vi "demo - math to file.vi"() -> ()   [LabVIEW 2024]
doc: "#vi_description \nPlots a polynomial equation to an XY graph and stores the values into a text file.\nThetic Engineering Ltd."
uses:
  <vilib>/Utility/sysdir.llb/System Directory Type.ctl
panel:
  in  "All data":dbl[][](array[numeric])=[[-10.0, -204.0, 492.55], [-9.0, -132.17359, 359.580355], [-8.0, -87.56192, 252.88208], [-7.0, -58.99533, 169.671655], [-6.0, -39.66976, 107.11768], [-5.0, -25.71875, 62.346875], [-4.0, -15.13824, 32.45008], [-3.0, -7.01377, 14.488255], [-2.0, -0.99968, 5.49848], [-1.0, 3.00009, 2.499955], [0.0, 5.0, 2.5], [1.0, 5.00011, 2.500055], [2.0, 3.00288, -0.49832], [3.0, -0.97003, -9.487445], [4.0, -6.81056, -27.44752], [5.0, -14.15625, -57.340625], [6.0, -22.07104, -102.10472], [7.0, -28.52447, -164.647645], [8.0, -29.61888, -247.84112], [9.0, -18.51421, -354.514745]]
  out "XY Graph":cluster{"x axis":dbl[], "plot 1":dbl[]}[](graph)
  out "Data written to":path
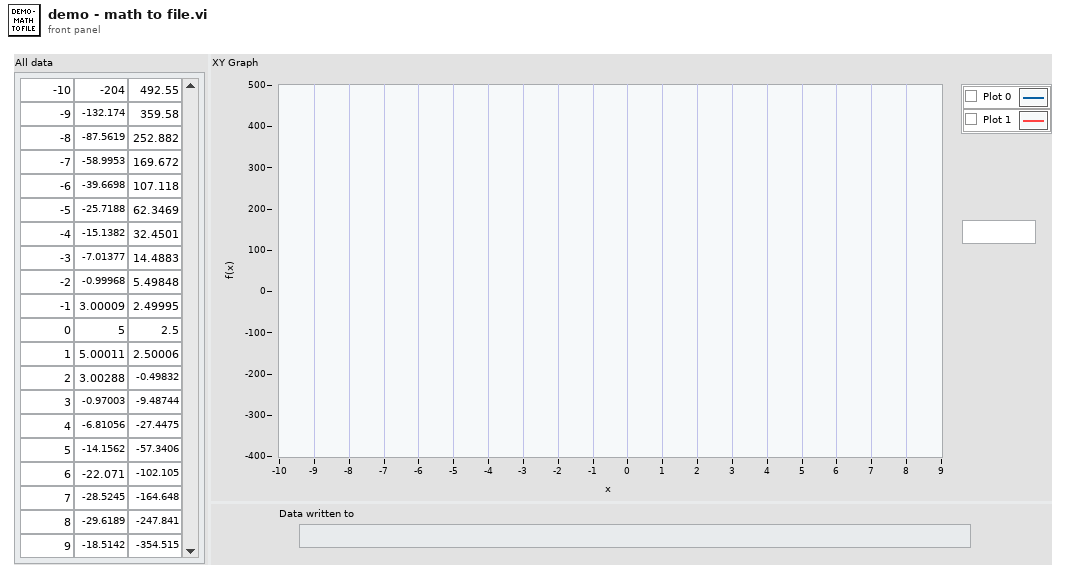
[diagram p1: front panel]
types:
  T1 = enum16{"open", "replace", "create", "open or create", "replace or create", "replace or create with confirmation"}
  T2 = typedef "System Directory Type.ctl" = i32
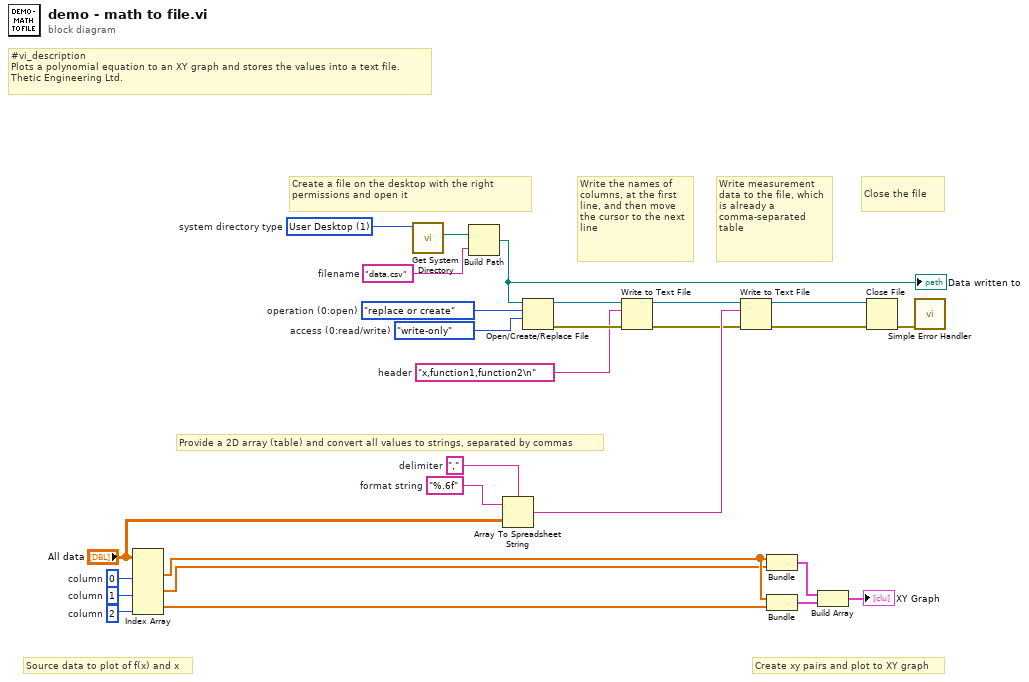
[diagram p0: block diagram]
diagram:
  w5 = 2  # column
  w6 = 1  # column
  w7 = 0  # column
  w9 = "x,function1,function2\n"  # header
  w11 = "data.csv"  # filename
  w12 = enum16{"read/write", "read-only", "write-only"}."write-only"  # access (0:read/write)
  w13 = T1."replace or create"  # operation (0:open)
  w15 = T2 1 items=["User Home"=0, "User Desktop"=1, "User Documents"=2, "User Application Data"=3, "User Preferences"=4, "User Temporary"=5, "Public Documents"=6, "Public Application Data"=7, "Public Preferences"=8, "Public Cache"=13, "System Core Libraries"=9, "System Installed Libraries"=10, "Application Files"=11, "Boot Volume Root"=12]  # system directory type
  w23 = ","  # delimiter
  w24 = "%.6f"  # format string
  # "Close the file"
  # "Write measurement data to the file, which is already a comma-separated table"
  # "Write the names of columns, at the first line, and then move the cursor to the next line"
  # "Create a file on the desktop with the right permissions and open it"
  # "Provide a 2D array (table) and convert all values to strings, separated by commas"
  # "Source data to plot of f(x) and x"
  # "#vi_description \nPlots a polynomial equation to an XY graph and stores the values into a text file.\nThetic Engineering Ltd."
  # "Create xy pairs and plot to XY graph"
  n1 = Index Array(array="All data", index (col) #1=w7, index (col) #2=w6, index (col) #3=w5) -> (element #1=w4:dbl[], element #2=w3:dbl[], element #3=w2:dbl[])  [unwired: 3 in]
  n2 = call <vilib>:"Get System Directory.vi"("system directory type"=w15) -> ("system directory"=w14:path)  [unwired: 10 in]
  n3 = Build Path(base path=w14, name or relative path=w11) -> (appended path=w8:path)
  "Data written to" <- w8
  n4 = Array To Spreadsheet String(delimiter (Tab)=w23, array="All data", 3:w24) -> (spreadsheet string=w22:string)
  n5 = Open/Create/Replace File(file path (use dialog)=w8, operation (0:open)=w13, access (0:read/write)=w12) -> (refnum out=w18:refnum<file>, error out=w19:errorcluster)  [unwired: 3 in, 1 out]
  n6 = Write to Text File(file (use dialog)=w18, text=w9, error in=w19) -> (refnum out=w20:refnum<file>, error out=w21:errorcluster)  [unwired: 1 in, 1 out]
  n7 = Write to Text File(file (use dialog)=w20, text=w22, error in=w21) -> (refnum out=w16:refnum<file>, error out=w17:errorcluster)  [unwired: 1 in, 1 out]
  n8 = Bundle("All data"=w4, "All data"=w3) -> (w27:cluster{"All data":dbl[], "All data":dbl[]})  [unwired: 1 in]
  n9 = Bundle("All data"=w4, "All data"=w2) -> (w26:cluster{"All data":dbl[], "All data":dbl[]})  [unwired: 1 in]
  n10 = Build Array(w27, w26) -> (→"XY Graph":cluster{"All data":dbl[], "All data":dbl[]}[])
  n11 = Close File(refnum=w16, error in=w17) -> (error out=w10:errorcluster)  [unwired: 1 out]
  n12 = call <vilib>:"Simple Error Handler.vi"("error in (no error)"=w10) -> ()  [unwired: 4 in, 5 out]
